vi "SessionManagementService ReserveSessions.vi"(8 "error in":errorcluster, 9 "timeout (ms)":i32=-1, 10 "Request Data":T4, 11 "gRPC ID":T6) -> (0 "error out":errorcluster, 2 "Response Data":T1, 3 "gRPC ID out":T6)   [LabVIEW 2020, in "Session Management Client_v1.lvlib"]
uses:
  Session Management Client_v1.lvlib
  <vilib>/gRPC/LabVIEW gRPC Library/Shared/grpcId.ctl
  RPC Messages/ni_measurementlink_sessionmanagement_v1_ReserveSessionsRequest.ctl
  RPC Messages/ni_measurementlink_PinMapContext.ctl
  RPC Messages/ni_measurementlink_sessionmanagement_v1_ReserveSessionsResponse.ctl
  RPC Messages/ni_measurementlink_sessionmanagement_v1_SessionInformation.ctl
  RPC Messages/ni_measurementlink_sessionmanagement_v1_Session.ctl
  3477ff3c-ac1a-41b2-98e0-1f89dff8fa77.vi
  <vilib>/gRPC/LabVIEW gRPC Library/Shared/TranslateGrpcError.vi
  <vilib>/gRPC/LabVIEW gRPC Library/Shared/Wait On Occurence.vi
  <vilib>/gRPC/LabVIEW gRPC Library/Server API/Server/Get Server DLL Path.vi
  <vilib>/Utility/error.llb/Error Cluster From Error Code.vi
  <vilib>/gRPC/LabVIEW gRPC Library/grpc-lvsupport-release.lvlib
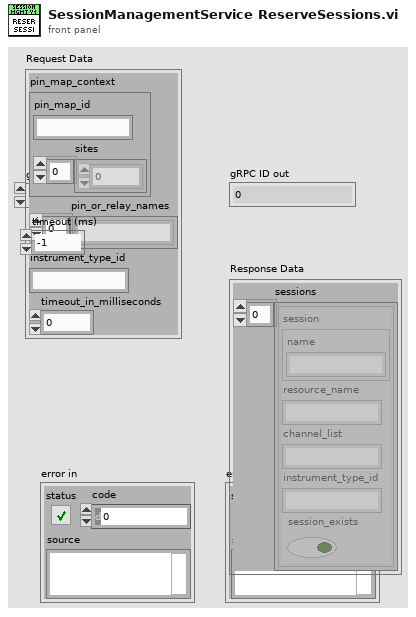
[diagram p1: front panel]
types:
  T1 = typedef "Session Management Client_v1.lvlib/ni_measurementlink_sessionmanagement_v1_ReserveSessionsResponse.ctl" = cluster{"sessions":T2[]}
  T2 = typedef "Session Management Client_v1.lvlib/ni_measurementlink_sessionmanagement_v1_SessionInformation.ctl" = cluster{"session":T3, "resource_name":string, "channel_list":string, "instrument_type_id":string, "session_exists":bool}
  T3 = typedef "Session Management Client_v1.lvlib/ni_measurementlink_sessionmanagement_v1_Session.ctl" = cluster{"name":string}
  T4 = typedef "Session Management Client_v1.lvlib/ni_measurementlink_sessionmanagement_v1_ReserveSessionsRequest.ctl" = cluster{"pin_map_context":T5, "pin_or_relay_names":string[], "instrument_type_id":string, "timeout_in_milliseconds":i32}
  T5 = typedef "Session Management Client_v1.lvlib/ni_measurementlink_PinMapContext.ctl" = cluster{"pin_map_id":string, "sites":i32[]}
  T6 = typedef "grpc-lvsupport-release.lvlib/grpcId.ctl" = u64
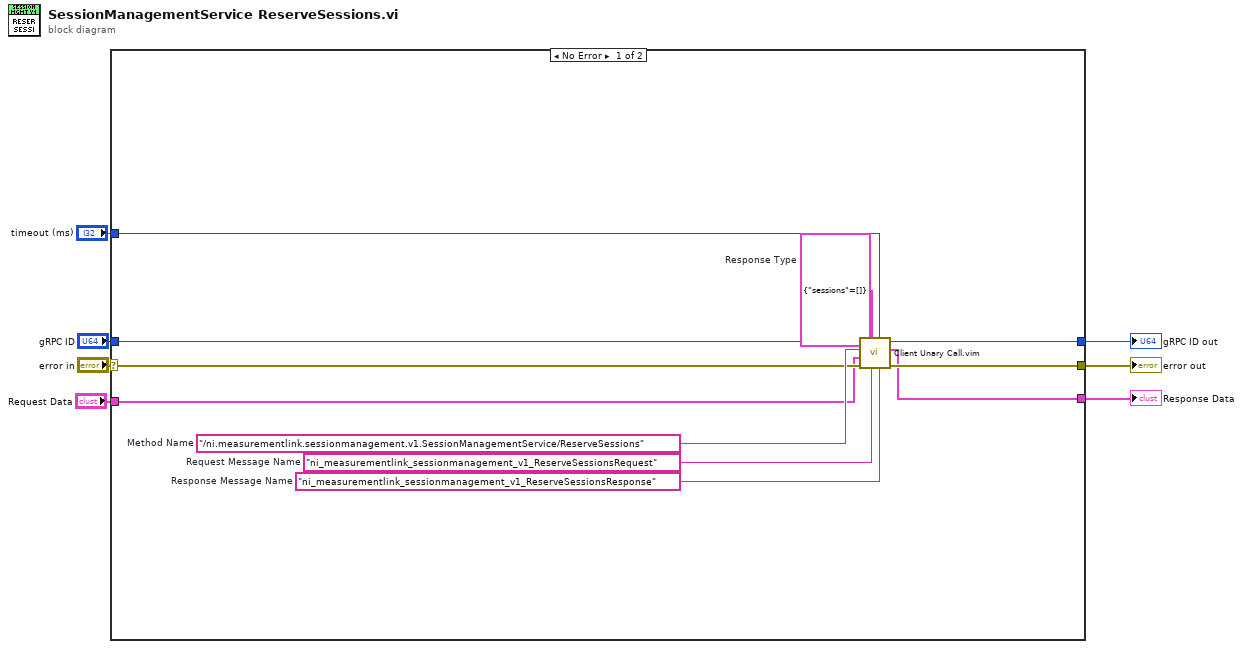
[diagram p0: block diagram]
diagram:
  n1 = case shown="No Error" "error in" {
    selector: "error in" -> [w14 w19]
    tunnel: [w13 w19] -> w6
    tunnel: "gRPC ID" -> [w12 w20]
    tunnel: [w11 w20] -> w4
    tunnel: "Request Data" -> [w10 _]
    tunnel: [w9 _] -> w2
    tunnel: "timeout (ms)" -> [w8 _]
    frame No Error {
      w15 = "ni_measurementlink_sessionmanagement_v1_ReserveSessionsResponse"  # Response Message Name
      w16 = "ni_measurementlink_sessionmanagement_v1_ReserveSessionsRequest"  # Request Message Name
      w17 = T1 {"sessions"=[]}  # Response Type
      w18 = "/ni.measurementlink.sessionmanagement.v1.SessionManagementService/ReserveSessions"  # Method Name
      n2 = call "Client Unary Call.vim"("Response Message Name"=w15, "timeout (ms)"=w8, "Request Message Name"=w16, "Response Type"=w17, "error in"=w14, "Request Data"=w10, "Method Name"=w18, "ClientID in"=w12) -> ("error out"=w13:errorcluster, "Response Data"=w9:T1, "ClientID out"=w11:u64)  [unwired: 1 in]
    }
    frame Error {
    }
  }
  "error out" <- w6
  "gRPC ID out" <- w4
  "Response Data" <- w2
